vi "Pcre2GetMatchOffsetsIndirect.vi"(8 "error in":errorcluster, 11 "pMatchData":u64 format="%.0x") -> (0 "error out":errorcluster, 1 "OffsetsPastMatch":i32[](array[numeric]), 2 "MatchOffsets":i32[](array[numeric]), 3 "pMatchData":u64 format="%.0x", 4 "pOvektor":u64 format="%.0x", 5 "SubstringCount":u32, 6 "pCode":u64 format="%.0x")   [LabVIEW 2021, in "libpcre2-8.lvlib"]
uses:
  libpcre2-8.lvlib
  Pcre2PatternInfoU32Data8.vi
  Pcre2ErrorNull.vi
  Pcre2FnkCallError.vi
  <vilib>/Utility/error.llb/Error Cluster From Error Code.vi
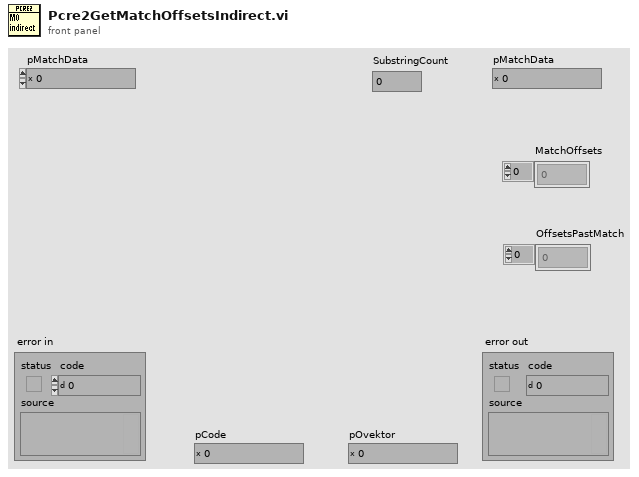
[diagram p1: front panel]
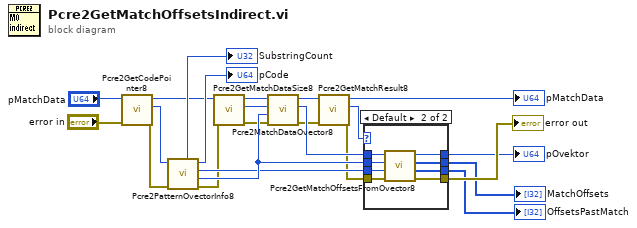
[diagram p0: block diagram]
diagram:
  n1 = call "Pcre2GetCodePointer8.vi"("error in"="error in", "pMatchData"="pMatchData") -> ("error out"=w20:errorcluster, "pCode"=w23:u64, "pMatchData"=w6:u64)  [unwired: 7 in]
  n2 = call "Pcre2PatternOvectorInfo8.vi"("error in"=w20, "pCode"=w23) -> ("error out"=w7:errorcluster, "OvectorSize"=w22:u64, "OvectorEntries"=w21:u32, "pCode"=→"pCode":u64, "SubstringCount"=→"SubstringCount":u32)  [unwired: 5 in]
  n3 = call "Pcre2GetMatchDataSize8.vi"("error in"=w7, "pMatchData"=w6) -> ("error out"=w10:errorcluster, "MatchDataSize"=w8:u64, "pMatchData"=w9:u64)  [unwired: 7 in]
  n4 = call "Pcre2MatchDataOvector8.vi"("error in"=w10, "OvectorSize"=w22, "MatchDataSize"=w8, "pMatchData"=w9) -> ("error out"=w2:errorcluster, "pOvector"=w11:u64, "pMatchData"=w5:u64)  [unwired: 5 in]
  n5 = call "Pcre2GetMatchResult8.vi"("error in"=w2, "pMatchData"=w5) -> ("error out"=w1:errorcluster, "MatchResult"=w3:i32, "pMatchData"=→"pMatchData":u64)  [unwired: 7 in]
  n6 = case shown="Default" w3 {
    tunnel: w22 -> [_ w33]
    tunnel: w21 -> [_ w32]
    tunnel: [w24 w31] -> w18
    tunnel: [_ w30] -> w16
    tunnel: [_ w29] -> w15
    tunnel: [w25 w28] -> w14
    tunnel: w11 -> [w25 w27]
    tunnel: w1 -> [w24 w26]
    frame ..0 {
    }
    frame Default {
      n7 = call "Pcre2GetMatchOffsetsFromOvector8.vi"("error in"=w26, "OvectorCount"=w32, "OvectorSize"=w33, "pOvector"=w27) -> ("error out"=w31:errorcluster, "OffsetsPastMatch"=w30:i32[], "MatchOffsets"=w29:i32[], "pOvector"=w28:u64)  [unwired: 4 in]
    }
  }
  "error out" <- w18
  "MatchOffsets" <- w15
  "OffsetsPastMatch" <- w16
  "pOvektor" <- w14
